vi "Get Time.vi"(8 "error in (no error)":errorcluster, 11 "Logging Thread in":refnum<class "Logging Thread.lvclass">) -> (0 "error out":errorcluster, 2 "time":dbl format="%.3fs", 3 "Logging Thread out":refnum<class "Logging Thread.lvclass">)   [LabVIEW 2021, in "DSF Core.lvlib" / "Logging Thread.lvclass"]
uses:
  Logging Thread.lvclass
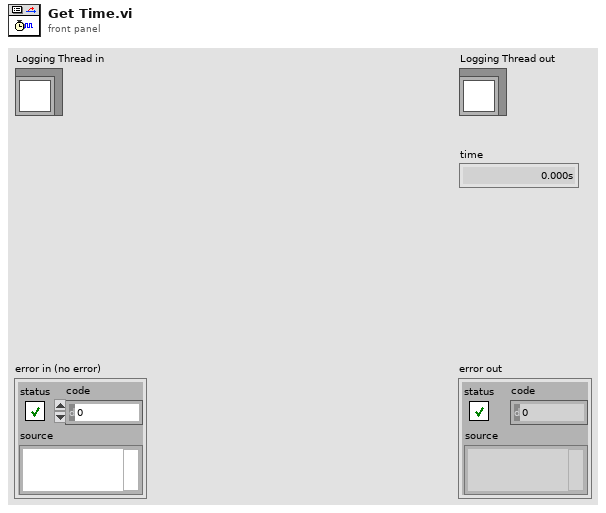
[diagram p1: front panel]
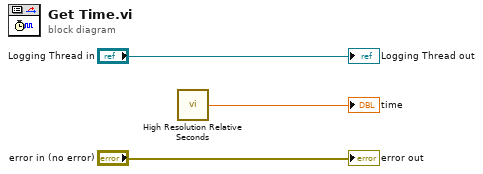
[diagram p0: block diagram]
diagram:
  n1 = call <vilib>:"High Resolution Relative Seconds.vi"() -> ("relative seconds"=→"time":dbl)
  "error out" <- "error in (no error)"
  "Logging Thread out" <- "Logging Thread in"
